vi "dfd_Render the Item of Difference Equation.vi"(4 "format control":T1={"function"="y", "variable"="n", "bracket"={"left"="(", "right"=")"}}, 5 "fonts input":T4(array[cluster]), 6 "alignment(left, top)":T3, 7 "format string":string="%#.4g", 9 "rect in":T2, 10 "coefficients array":dbl[](array[numeric]), 11 "picture in":picture) -> (1 "rect out":T2, 3 "picture out":picture)   [LabVIEW 2017, in "NI_DigFilter_Process.lvlib"]
uses:
  <vilib>/addons/Digital Filter Design/NI_DigFilter_Process.lvlib
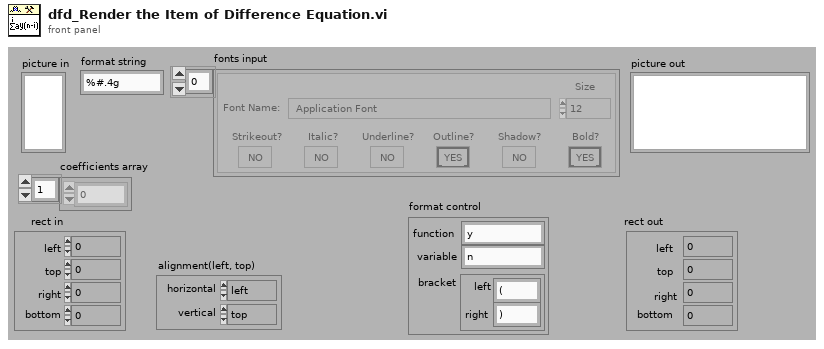
[diagram p1: front panel]
types:
  T1 = cluster{"function":string, "variable":string, "bracket":cluster{"left":string, "right":string}}
  T2 = cluster{"left":i16, "top":i16, "right":i16, "bottom":i16}
  T3 = cluster{"horizontal":enum16{"left", "center", "right"}, "vertical":enum16{"top", "center", "bottom"}}
  T4 = cluster{"Font Name:":string, "Size":i16, "Strikeout?":bool, "Italic?":bool, "Underline?":bool, "Outline?":bool, "Shadow?":bool, "Bold?":bool}[]
  T5 = cluster{"Font Name:":string, "Size":i16, "Strikeout?":bool, "Italic?":bool, "Underline?":bool, "Outline?":bool, "Shadow?":bool, "Bold?":bool}
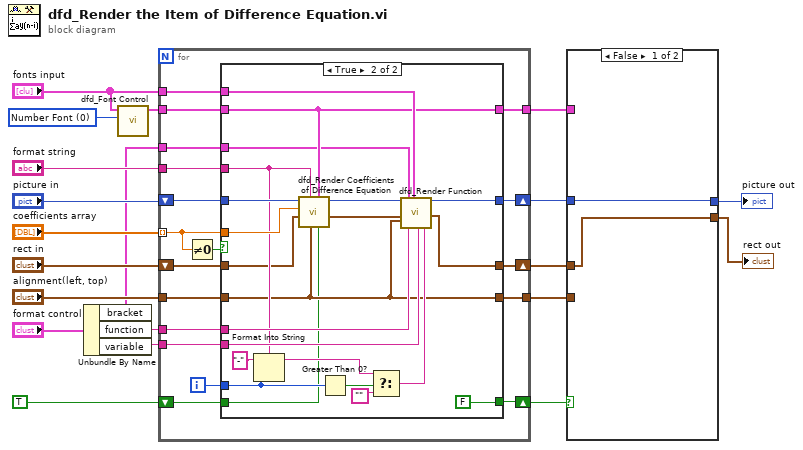
[diagram p0: block diagram]
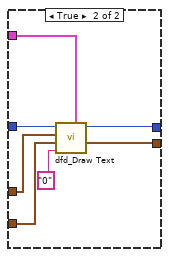
[diagram p2: hidden frame]
diagram:
  w5 = u16 0 items=["Number Font", "Variable Font", "Script Font"] ("Tpye")
  n1 = Unbundle By Name("format control") -> ("bracket"=w1:cluster{"left":string, "right":string}, "function"=w3:string, "variable"=w2:string)
  n2 = call <vilib>:"dfd_Font Control.vi"("tpye"=w5, "fonts input"="fonts input") -> ("font output"=w17:T5)  [unwired: 9 out]
  n3 = for {
    tunnel: "coefficients array" -> [w36] mode=indexing
    shift-right: [w31] -> w12
    shift-left: TRUE ("first non-zero coefficient") -> [w32]
    shift-right: [w37] -> w10
    shift-left: "picture in" -> [w38]
    tunnel: "fonts input" -> [w34]
    tunnel: w17 -> [w33]
    tunnel: "format string" -> [w30]
    tunnel: "alignment(left, top)" -> [w28]
    tunnel: w3 -> [w27]
    tunnel: w2 -> [w26]
    shift-right: [w25] -> w9
    shift-left: "rect in" -> [w29]
    tunnel: [w23] -> w11
    tunnel: [w22] -> w8
    tunnel: w1 -> [w21]
    i -> [w24]
    n4 = Not Equal To 0?(x=w36) -> (x != 0?=w35:bool)
    n5 = case shown="True" w35 {
      tunnel: w36 -> [_ w65]
      tunnel: w38 -> [w43 w64]
      tunnel: [w43 w62] -> w37
      tunnel: w34 -> [_ w61]
      tunnel: w33 -> [w40 w49]
      tunnel: w32 -> [w42 w45]
      tunnel: [w42 FALSE] -> w31
      tunnel: w30 -> [_ w56]
      tunnel: w29 -> [w41 w47]
      tunnel: w28 -> [w39 w48]
      tunnel: w27 -> [_ w58]
      tunnel: w26 -> [_ w57]
      tunnel: [w41 w46] -> w25
      tunnel: w24 -> [_ w54]
      tunnel: [w40 w49] -> w23
      tunnel: [w39 w48] -> w22
      tunnel: w21 -> [_ w44]
      frame False {
      }
      frame True {
        n6 = Format Into String(format string=w56, initial string="-", w54) -> (resulting string=w52:string)  [unwired: 1 in, 1 out]
        n7 = call <vilib>:"dfd_Render Coefficients of Difference Equation.vi"("first non-zero coefficient"=w45, "[user-specified font]"=w49, "alignment(left, top)"=w48, "format string"=w56, "rect in"=w47, "coefficient"=w65, "picture in"=w64) -> ("rect out"=w59:T2, "picture out"=w63:picture)  [unwired: 3 out]
        n8 = Greater Than 0?(x=w54) -> (x > 0?=w53:bool)
        n9 = Select(t=w52, s=w53, f="") -> (s? t:f=w51:string)
        n10 = call <vilib>:"dfd_Render Function.vi"("picture"=w63, "rect in"=w59, "alignment(left, top)"=w48, "bracket"=w44, "function name"=w58, "fonts input"=w61, "variable"=w57, "modification"=w51) -> ("new picture"=w62:picture, "rect out"=w46:T2)  [unwired: 2 in, 8 out]
      }
    }
  }
  n11 = case shown="False" w12 {
    tunnel: w11 -> [_ w74]
    tunnel: w10 -> [w67 w73]
    tunnel: w9 -> [w66 w72]
    tunnel: w8 -> [_ w71]
    tunnel: [w67 w70] -> w7
    tunnel: [w66 w68] -> w6
    frame False {
    }
    frame True {
      n12 = call <vilib>:"dfd_Draw Text.vi"("font input"=w74, "text"="0", "alignment(left, top)"=w71, "rect in"=w72, "picture in"=w73) -> ("rect out"=w68:T2, "picture out"=w70:picture)  [unwired: 3 in, 2 out]
    }
  }
  "picture out" <- w7
  "rect out" <- w6
